vi "DSF.Engine.Plugin.Set Timing.vi"(10 "Timing":refnum<class "DSF.Shared.Timing.lvclass">, 11 "Plugin in":refnum<class "Plugin.lvclass">) -> (3 "Plugin out":refnum<class "Plugin.lvclass">)   [LabVIEW 2016, in "DSF.Engine.lvlib" / "Plugin.lvclass"]
uses:
  Plugin.lvclass
  Shared/Classes/Timing/DSF.Shared.Timing.lvclass
  Plugin.lvclass/Plugin.ctl
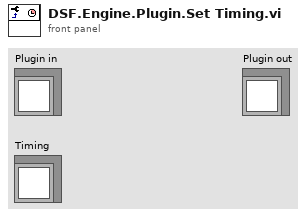
[diagram p1: front panel]
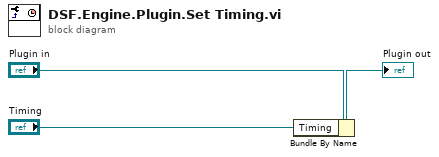
[diagram p0: block diagram]
diagram:
  n1 = Bundle By Name(cluster="Plugin in", "Timing"="Timing") -> (→"Plugin out":refnum<class "Plugin.lvclass">)
